vi "DAQmx Create Channel (AO-FuncGen).vi"(0 "task in":refnum<k21>, 1 "frequency":dbl=1000.0 format="%.2f", 2 "amplitude":dbl=5.0 format="%.2f", 3 "offset":dbl format="%.2f", 5 "physical channels":tag, 7 "name to assign":string, 9 "type":i32(ring)=14751 items=["Sine"=14751, "Triangle"=14752, "Square"=14753, "Sawtooth"=14754], 11 "error in":errorcluster) -> (4 "task out":refnum<k21>, 15 "error out":errorcluster)   [LabVIEW 2018]
doc: "Creates a channel for continually generating a waveform on the selected physical channel."
uses:
  nilvaiu.dll
panel:
  # "output limits"
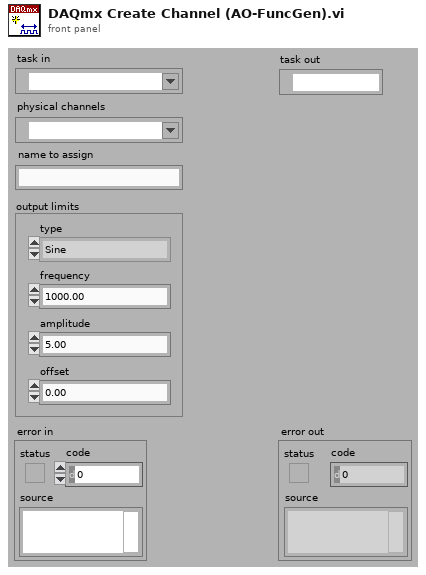
[diagram p1: front panel]
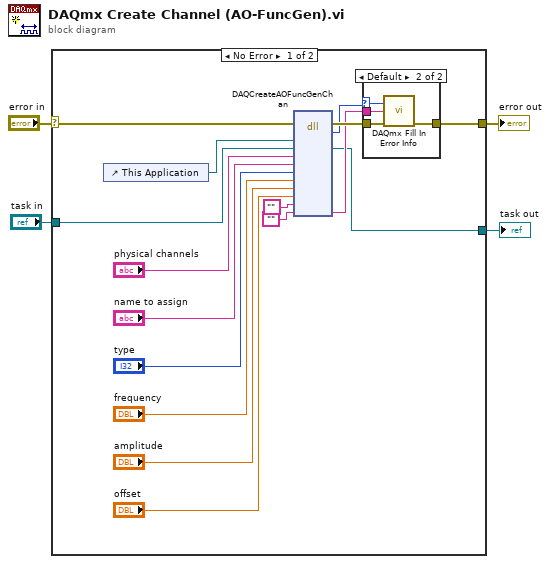
[diagram p0: block diagram]
diagram:
  n1 = case shown="No Error" "error in" {
    selector: "error in" -> [w7 w26]
    tunnel: [w17 w26] -> w4
    tunnel: "task in" -> [w9 w27]
    tunnel: [w8 w27] -> w2
    frame No Error {
      n2 = control-ref of="This Application"() -> (w20:refnum<vi>)
      n3 = dll-call lib="nilvaiu.*" fn="DAQCreateAOFuncGenChan"(error in=w7, "lvAppRef"=w20, "refObjPtr"=w9, "physicalChannelName"="physical channels", "channelNameIn"="name to assign", "type"="type", "frequency"="frequency", "amplitude"="amplitude", "offset"="offset", "channelNamesOut"="", "extendedErrorInfo"="") -> (error out=w18:errorcluster, "return type"=w6:i32, "refObjPtr"=w8:refnum<k21>, "extendedErrorInfo"=w12:string)  [unwired: 10 in, 1 out]
      n4 = case shown="Default" w6 {
        selector: w6 -> [_ w22]
        tunnel: w18 -> [w21 w25]
        tunnel: [w21 w24] -> w17
        tunnel: w12 -> [_ w23]
        frame 0 {
        }
        frame Default {
          n5 = call "DAQmx Fill In Error Info.vi"("status code"=w22, "extended error info"=w23, "error in"=w25) -> ("error out"=w24:errorcluster)  [unwired: 1 in, 11 out]
        }
      }
    }
    frame Error {
    }
  }
  "error out" <- w4
  "task out" <- w2
